vi "List tables.vi"(8 "error in (no error)":errorcluster, 11 "database":string) -> (0 "error out":errorcluster, 3 "tables":string[](array[string]))   [LabVIEW 2016, in "氨氮.lvlib"]
uses:
  <vilib>/Utility/sysdir.llb/System Directory Type.ctl
  <vilib>/addons/database/Connection.llb/DB Tools Open Connec (String).vi
  <vilib>/addons/database/NI_Database_API.lvlib
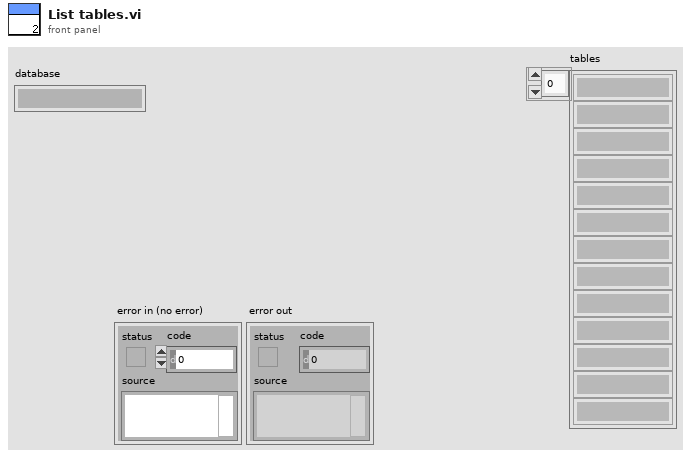
[diagram p1: front panel]
types:
  T1 = typedef "System Directory Type.ctl" = i32
  T2 = typedef "NI_Database_API.lvlib/Conn ObjectReference.ctl" = refnum<k1>
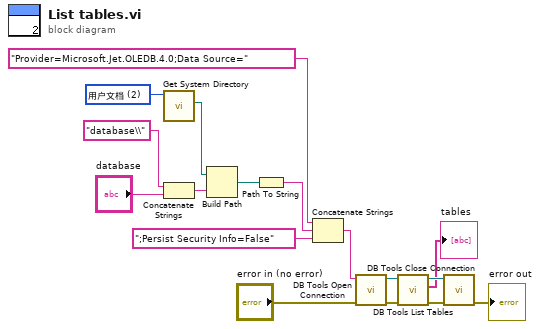
[diagram p0: block diagram]
diagram:
  w11 = T1 2 items=["用户目录"=0, "用户桌面"=1, "用户文档"=2, "用户应用程序数据"=3, "用户设置"=4, "用户临时目录"=5, "公共文档"=6, "公共应用程序数据"=7, "公共设置"=8, "公共缓存"=13, "系统核心库"=9, "系统安装库"=10, "应用程序文件"=11, "启动盘根目录"=12] ("system directory type")
  n1 = call <vilib>:"Get System Directory.vi"("system directory type"=w11) -> ("system directory"=w9:path)  [unwired: 10 in]
  n2 = Concatenate Strings("database\\" ("condition"), "database") -> (w3:string)
  n3 = Build Path(base path=w9, name or relative path=w3) -> (appended path=w8:path)
  n4 = Path To String(path=w8) -> (string=w7:string)
  n5 = Concatenate Strings("Provider=Microsoft.Jet.OLEDB.4.0;Data Source=" ("condition"), w7, ";Persist Security Info=False" ("condition")) -> (w5:string)
  n6 = call-poly <vilib>:"DB Tools Open Connection.vi"("error in (no error)"="error in (no error)", "connection information"=w5) -> ("error out"=w15:errorcluster, "connection reference"=w17:T2)  [unwired: 6 in]
  n7 = call <vilib>:"DB Tools List Tables.vi"("error in (no error)"=w15, "connection reference"=w17) -> ("error out"=w14:errorcluster, "tables"=→"tables":string[], "connection reference out"=w16:T2)  [unwired: 3 in]
  n8 = call <vilib>:"DB Tools Close Connection.vi"("error in (no error)"=w14, "connection reference"=w16) -> ("error out"=→"error out":errorcluster)  [unwired: 5 in]
